vi "GVSView Queue.vi"() -> ()   [LabVIEW 2013]
uses:
  GVSView Global.vi
  SubVI/GVSMain Sub Window Global.vi
panel:
  in  "bVIRefRemove":bool=TRUE
  in  "ResultInCurLibrary":T1={"bResult"=TRUE, "SData_Out"="", "pVIRef_Out"=refnum, "pRefList_Out"=[]}
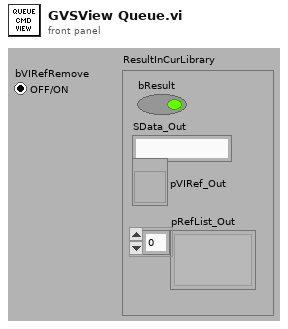
[diagram p1: front panel]
types:
  T1 = cluster{"bResult":bool, "SData_Out":string, "pVIRef_Out":refnum<vi>, "pRefList_Out":variant[]}
  T2 = cluster{"sCmdType":string, "nIDView":i32, "sAction":string, "sData":string, "sOption":string, "nData":i32, "nOption":i32, "pVIRef":refnum<vi>, "pSPRef":refnum<vi>, "bWaitRef":refnum<vi>, "Result":variant}[]
  T3 = cluster{"sCmdType":string, "nIDView":i32, "sAction":string, "sData":string, "sOption":string, "nData":i32, "nOption":i32, "pVIRef":refnum<vi>, "pSPRef":refnum<vi>, "bWaitRef":refnum<vi>, "Result":variant}
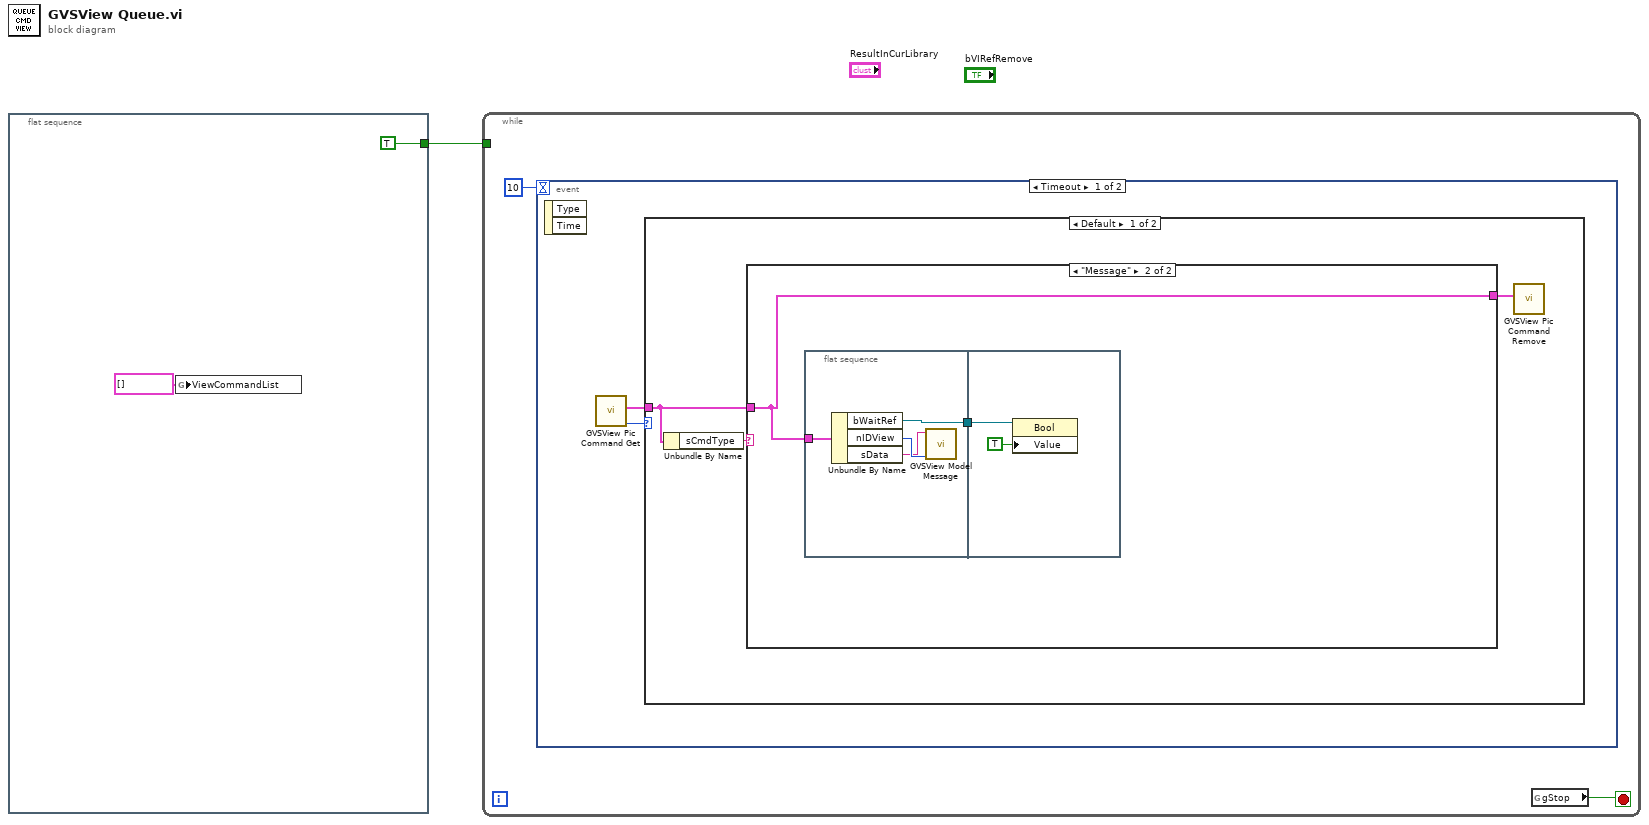
[diagram p0: block diagram]
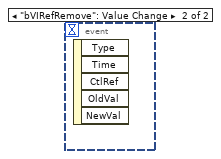
[diagram p4: hidden frame]
diagram:
  n1 = flat-sequence {
    tunnel: [TRUE] -> w1
    frame #0 {
      n2 = global write "GVSView Global.vi" "ViewCommandList"(T2 [] ("ViewCommandList")) -> ()
    }
  }
  n3 = while {
    tunnel: w1 -> [_]
    stop <- w4 stop-if-true
    n4 = event shown="[0] Timeout" {
      selector: _ -> [_ _]
      dyn-events: _ -> [_ _]
      timeout: 10 -> [_ _]
      event Timeout {
        n5 = event-data() -> ()  [unwired: 1 in, 2 out]
        n6 = call "GVSView Pic  Command Get.vi"() -> ("nData_Out"=w7:i32, "cCommand_Out"=w6:T3)  [unwired: 10 in]
        n7 = case shown="Default" w7 {
          tunnel: w6 -> [w9 _]
          frame Default {
            n8 = Unbundle By Name(w9) -> ("sCmdType"=w10:string)
            n9 = case shown="\"Message\"" w10 {
              tunnel: w9 -> [w11 w12]
              tunnel: [w11 w12] -> w8
              frame Default {
              }
              frame "Message" {
                n10 = flat-sequence {
                  tunnel: w12 -> [w15]
                  tunnel: [w14] -> w13
                  tunnel: w13 -> [w18]
                  frame #0 {
                    n11 = Unbundle By Name(w15) -> ("bWaitRef"=w14:refnum<vi>, "nIDView"=w17:i32, "sData"=w16:string)
                    n12 = call "GVSView Model Message.vi"("nData"=w17, "sMsgData"=w16) -> ()  [unwired: 7 in, 3 out]
                  }
                  frame #1 {
                    n13 = property class="Bool"(reference=w18, "Value"=TRUE) -> ()  [unwired: 1 in, 2 out]
                  }
                }
              }
            }
            n14 = call "GVSView Pic Command Remove.vi"("cCommand"=w8) -> ()  [unwired: 11 in]
          }
          frame 0 {
          }
        }
      }
      event "bVIRefRemove": Value Change {
        n15 = event-data() -> ()  [unwired: 1 in, 5 out]
      }
    }
    n16 = global read "GVSMain Sub Window Global.vi" "gStop"() -> (w4:bool)
  }
